vi "isReservedCharacter.vi"(11 "character":string) -> (2 "sub delimiter":bool, 3 "general delimiter":bool)   [LabVIEW 2013, in "openURI.lvlib"]
uses:
  openURI.lvlib
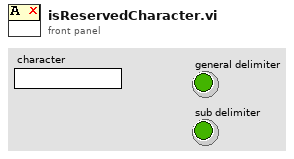
[diagram p1: front panel]
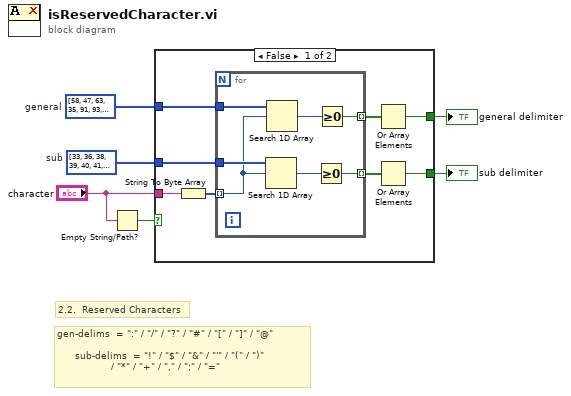
[diagram p0: block diagram]
diagram:
  w1 = u8[] [33, 36, 38, 39, 40, 41, 42, 43, 44, 59, 61]  # sub
  w2 = u8[] [58, 47, 63, 35, 91, 93, 64]  # general
  # "2.2.  Reserved Characters"
  # "gen-delims  = \":\" / \"/\" / \"?\" / \"#\" / \"[\" / \"]\" / \"@\"\n\n      sub-delims  = \"!\" / \"$\" / \"&\" / \"'\" / \"(\" / \")\"\n                  / \"*\" / \"+\" / \",\" / \";\" / \"=\""
  n1 = Empty String/Path?(string/path="character") -> (empty?=w3:bool)
  n2 = case shown="False" w3 {
    tunnel: "character" -> [w14 _]
    tunnel: [w12 _] -> w5
    tunnel: [w11 _] -> w4
    tunnel: w2 -> [w10 _]
    tunnel: w1 -> [w9 _]
    frame False {
      n3 = String To Byte Array(string=w14) -> (unsigned byte array=w13:u8[])
      n4 = for {
        tunnel: w13 -> [w19] mode=indexing
        tunnel: w10 -> [w21]
        tunnel: w9 -> [w20]
        tunnel: [w16] -> w8 mode=indexing
        tunnel: [w15] -> w7 mode=indexing
        n5 = Search 1D Array(1D array=w20, element=w19) -> (index of element=w17:i32)  [unwired: 1 in]
        n6 = Search 1D Array(1D array=w21, element=w19) -> (index of element=w18:i32)  [unwired: 1 in]
        n7 = Greater Or Equal To 0?(x=w17) -> (x >= 0?=w15:bool)
        n8 = Greater Or Equal To 0?(x=w18) -> (x >= 0?=w16:bool)
      }
      n9 = Or Array Elements(Boolean array=w8) -> (logical OR=w12:bool)
      n10 = Or Array Elements(Boolean array=w7) -> (logical OR=w11:bool)
    }
    frame True {
    }
  }
  "general delimiter" <- w5
  "sub delimiter" <- w4
